vi "Read Pref.vi"() -> ()   [LabVIEW 2020, in "Pref Tests.lvlib"]
uses:
  Pref Tests.lvlib
  User Prefs/PrefsDB/PrefsDB.lvclass
  User Prefs/Pref Group/Pref Group.lvclass
panel:
  out "error out":errorcluster
  out "Value":string
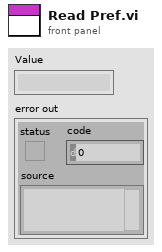
[diagram p1: front panel]
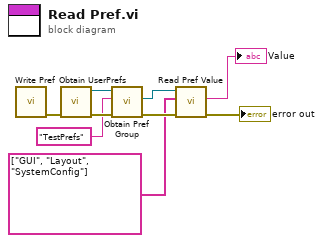
[diagram p0: block diagram]
diagram:
  n1 = call "Write Pref.vi"() -> ("error out"=w6:errorcluster)  [unwired: 11 in]
  n2 = call "Obtain UserPrefs.vi"("error in (no error)"=w6) -> ("error out"=w9:errorcluster, "PrefsDB out"=w8:refnum<class "PrefsDB.lvclass">)  [unwired: 9 in]
  n3 = call "Obtain Pref Group.vi"("error in (no error)"=w9, "Group"="TestPrefs", "PrefsDB in"=w8) -> ("error out"=w5:errorcluster, "Pref Group"=w4:refnum<class "Pref Group.lvclass">)  [unwired: 6 in, 1 out]
  n4 = call "Read Pref Value.vi"("error in (no error)"=w5, "Pref Hierarchy"=string[] ["GUI", "Layout", "SystemConfig"], "Pref Group in"=w4) -> ("error out"=→"error out":errorcluster, "Value"=→"Value":string)  [unwired: 6 in, 1 out]
